vi "UI Set DisableState.vi"(7 "Enable?":bool=TRUE, 8 "error in (no error)":errorcluster, 11 "UI.Refs":T1) -> (0 "error out":errorcluster, 3 "UI.Refs out":T1)   [LabVIEW 2019, in "Control Workspace Tool.lvlib"]
uses:
  Control Workspace Tool.lvlib
  Types/UI Refs.ctl
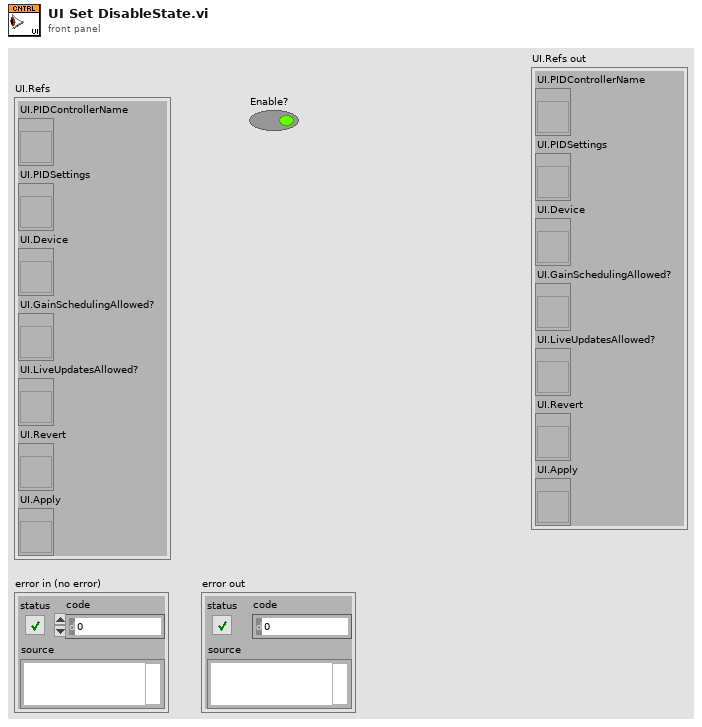
[diagram p1: front panel]
types:
  T1 = typedef "Control Workspace Tool.lvlib/UI Refs.ctl" = cluster{"UI.PIDControllerName":refnum<vi>, "UI.PIDSettings":refnum<vi>, "UI.Device":refnum<vi>, "UI.GainSchedulingAllowed?":refnum<vi>, "UI.LiveUpdatesAllowed?":refnum<vi>, "UI.Revert":refnum<vi>, "UI.Apply":refnum<vi>}
  T2 = enum8{"Enabled", "Disabled", "Disabled and Grayed Out"}
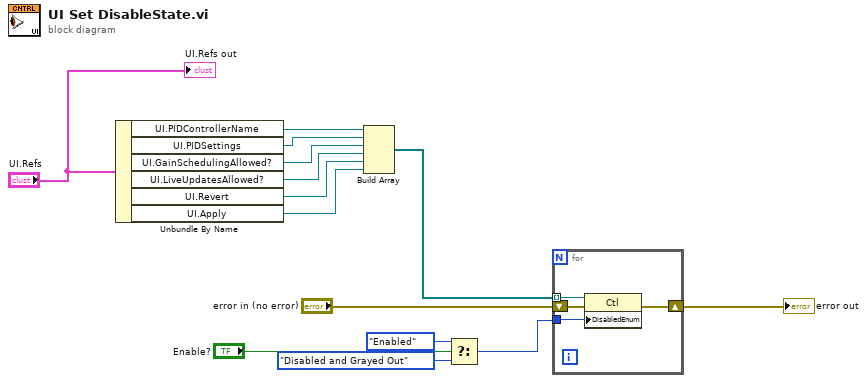
[diagram p0: block diagram]
diagram:
  n1 = Unbundle By Name("UI.Refs") -> ("UI.PIDControllerName"=w13:refnum<vi>, "UI.PIDSettings"=w12:refnum<vi>, "UI.GainSchedulingAllowed?"=w11:refnum<vi>, "UI.LiveUpdatesAllowed?"=w10:refnum<vi>, "UI.Revert"=w9:refnum<vi>, "UI.Apply"=w8:refnum<vi>)
  n2 = Build Array(w13, w12, w11, w10, w9, w8) -> (w1:refnum<vi>[])
  n3 = Select(t=T2."Enabled" ("Disabled"), s="Enable?", f=T2."Disabled and Grayed Out" ("Disabled")) -> (s? t:f=w4:T2)
  n4 = for {
    tunnel: w1 -> [w18] mode=indexing
    shift-right: [w16] -> w2
    shift-left: "error in (no error)" -> [w17]
    tunnel: w4 -> [w15]
    n5 = property class="Ctl"(reference=w18, error in=w17, "DisabledEnum"=w15) -> (error out=w16:errorcluster)  [unwired: 1 out]
  }
  "error out" <- w2
  "UI.Refs out" <- "UI.Refs"
